vi "S3Acq_fource_ai0.vi"() -> ()   [LabVIEW 2012]
doc: "I. Description:\nThis example demonstrates how to take a single Measurement (Sample) from an Analog Input Channel.\n\nII. Instructions for Running:\n1. Select the Physical Channel to correspond to where your signal is input on the DAQ device.\n2. Enter the Minimum and Maximum Voltage Ranges\nNote: For better accuracy try to match the Input Ranges to the expected voltage level of the measured signal.\nNote: Use the Gen Voltage Update example to provide a signal on your DAQ device to measure.\n\nIII. Block Diagram Steps:\n1. Create an Analog Input Voltage Channel.\n2. Use the Read VI to Measure 1 Sample from 1 Channel on the Data\nAcquisition Card. Set a timeout so an error is returned if the sample\nis not returned in the specified time limit\n3. Call the Clear Task VI to clear the Task.\n4. Use the popup dialog box to display an error if any.\n\nIV. I/O Connections Overview:\nMake sure your signal input terminal matches the Physical Channel I/O Control."
uses:
  <vilib>/Utility/error.llb/DialogType.ctl
  <vilib>/DAQmx/read.llb/DAQmx Read (Analog DBL 1Chan 1Samp).vi
  <vilib>/DAQmx/create/channels.llb/DAQmx Create Channel (AI-Voltage-Basic).vi
  2015myGlobal 1.vi
  <vilib>/DAQmx/miscellaneous.llb/DAQmx Fill In Error Info.vi
panel:
  in  "Sample Rate":dbl=50.0
  out "Waveform Chart":dbl(graph)
  in  "stop":bool
  out "Load Cell":dbl(knob) caption="Measurement" scale=-15.0..20.0
  in  "Maximum Value":dbl=10.0 format="%.2f"
  in  "Minimum Value":dbl=-10.0 format="%0.2f"
  in  "Physical Channel":tag="Dev2/ai0"
  # "For instructions, select Help>>Show Context Help"
  # "Channel Parameters"
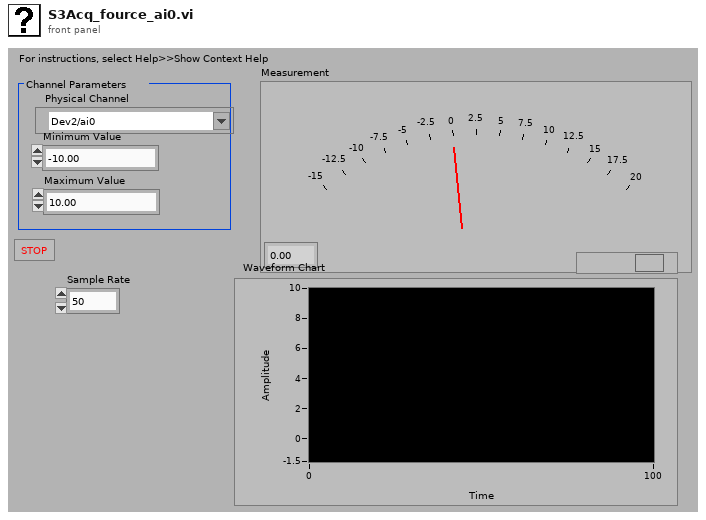
[diagram p1: front panel]
types:
  T1 = typedef "DialogType.ctl" = u16
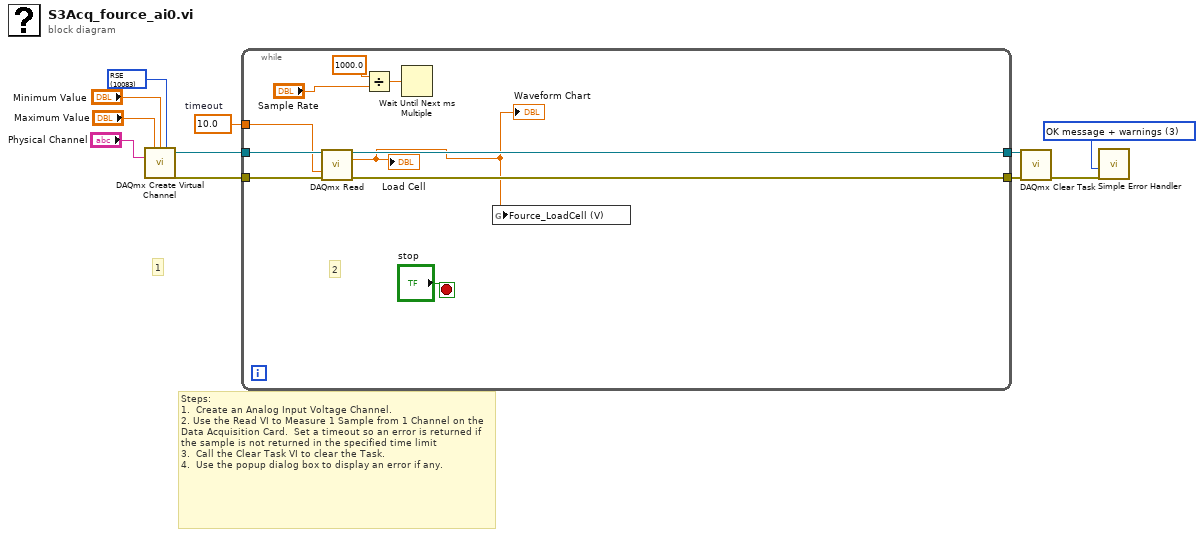
[diagram p0: block diagram]
diagram:
  w1 = 10083 items=["default"=-1, "RSE"=10083, "NRSE"=10078, "Differential"=10106, "Pseudodifferential"=12529] ("input terminal configuration")
  w5 = T1 3 items=["no dialog", "OK message", "continue or stop message", "OK message + warnings", "continue/stop + warnings"] ("type of dialog (OK msg:1)")
  w6 = 10.0  # timeout
  # "Steps: \n1.  Create an Analog Input Voltage Channel. \n2. Use the Read VI to Measure 1 Sample from 1 Channel on the Data Acquisition Card.  Set a timeout so an error is returned if the sample is not returned in the specified time limit\n3.  Call the Clear Task VI to clear the Task.\n4.  Use the popup dialog box to display an error if any."
  # "1"
  n1 = call-poly <vilib>:"DAQmx Create Virtual Channel.vi"("maximum value"="Maximum Value", "minimum value"="Minimum Value", "input terminal configuration"=w1, "physical channels"="Physical Channel") -> ("task out"=w8:refnum<k21>, "error out"=w7:errorcluster)  [unwired: 10 in]
  n2 = while {
    tunnel: w8 -> [w21]
    tunnel: w7 -> [w20]
    tunnel: w6 -> [w19]
    tunnel: [w18] -> w4
    tunnel: [w17] -> w3
    stop <- "stop" stop-if-true
    # "2"
    n3 = call-poly <vilib>:"DAQmx Read.vi"("task/channels in"=w21, "timeout"=w19, "error in"=w20) -> ("task out"=w18:refnum<k21>, "data"=w12:dbl, "error out"=w17:errorcluster)  [unwired: 10 in]
    "Load Cell" <- w12
    "Waveform Chart" <- w12
    n4 = Divide(x=1000.0, y="Sample Rate") -> (x/y=w15:dbl)
    n5 = Wait Until Next ms Multiple(millisecond multiple=w15) -> ()  [unwired: 1 out]
    n6 = global write "2015myGlobal 1.vi" "Fource_LoadCell (V)"(w12) -> ()
  }
  n7 = call <vilib>:"DAQmx Clear Task.vi"("task in"=w4, "error in"=w3) -> ("error out"=w2:errorcluster)  [unwired: 13 in]
  n8 = call <vilib>:"Simple Error Handler.vi"("type of dialog (OK msg:1)"=w5, "error in (no error)"=w2) -> ()  [unwired: 3 in, 5 out]
